vi "Get VI Name.vi"(1 "VI Refnum":refnum<vi>) -> (0 "VI Name":string)   [LabVIEW 2020, in "QTab.lvlib" / "QTab Class.lvclass"]
uses:
  QTab Class.lvclass
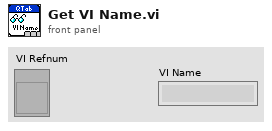
[diagram p1: front panel]
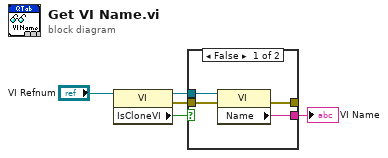
[diagram p0: block diagram]
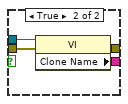
[diagram p2: hidden frame]
diagram:
  n1 = property class="VI"(reference="VI Refnum") -> (reference out=w2:refnum<vi>, error out=w3:errorcluster, "IsCloneVI"=w4:bool)  [unwired: 1 in]
  n2 = case shown="False" w4 {
    tunnel: w3 -> [w9 w13]
    tunnel: w2 -> [w8 w12]
    tunnel: [w7 w11] -> w1
    tunnel: [w6 w10] -> _
    frame False {
      n3 = property class="VI"(reference=w8, error in=w9) -> (error out=w6:errorcluster, "Name"=w7:string)  [unwired: 1 out]
    }
    frame True {
      n4 = property class="VI"(reference=w12, error in=w13) -> (error out=w10:errorcluster, "Clone Name"=w11:string)  [unwired: 1 out]
    }
  }
  "VI Name" <- w1
